vi "Rig_Create.vi"(8 "error in (no error)":errorcluster, 10 "ID":string, 11 "reference in":refnum<class "Rig.lvclass">) -> (0 "error out":errorcluster, 3 "reference out":refnum<class "Rig.lvclass">)   [LabVIEW 2020, in "Rig.lvclass"]
uses:
  Rig.lvclass
  C:/Projects/DesignPatterns/VisitorPattern/Equipment_class/Equipment.lvclass
  Equipment_class/Equipment.lvclass
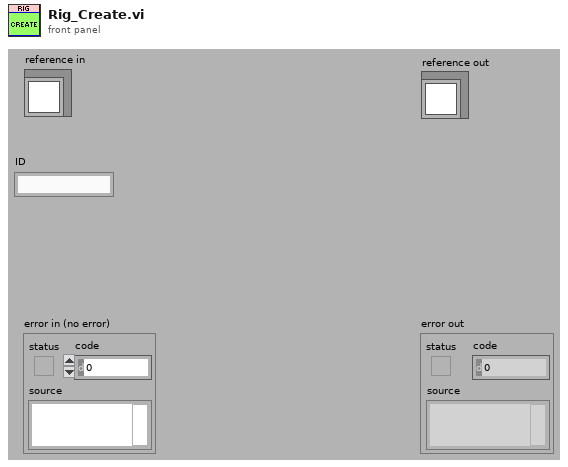
[diagram p1: front panel]
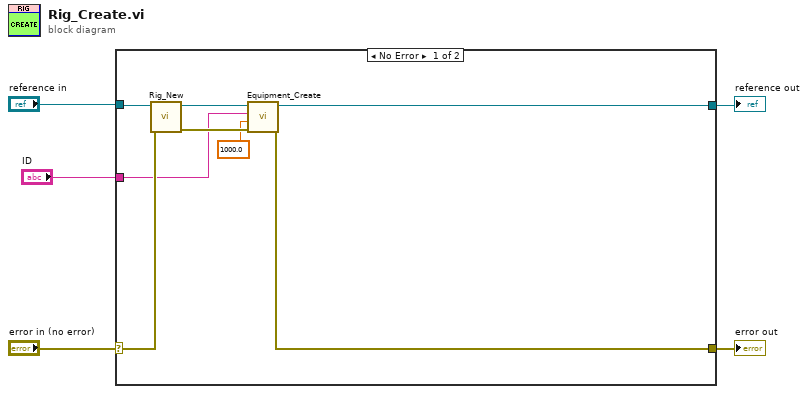
[diagram p0: block diagram]
diagram:
  n1 = case shown="No Error" "error in (no error)" {
    selector: "error in (no error)" -> [w10 w15]
    tunnel: [w7 w15] -> w4
    tunnel: "reference in" -> [w12 w14]
    tunnel: [w9 w14] -> w2
    tunnel: "ID" -> [w8 _]
    frame No Error {
      n2 = call "Rig_New.vi"("error in (no error)"=w10, "reference in"=w12) -> ("error out"=w11:errorcluster, "reference out"=w13:refnum<class "Rig.lvclass">)  [unwired: 6 in, 2 out]
      n3 = call "Equipment_Create.vi"("error in (no error)"=w11, "Cost"=1000.0, "ID"=w8, "reference in"=w13) -> ("error out"=w7:errorcluster, "reference out"=w9:refnum<class "Rig.lvclass">)  [unwired: 6 in]
    }
    frame Error {
    }
  }
  "error out" <- w4
  "reference out" <- w2
